vi "IMAQ Readfile.vi"   [LabVIEW 2017]
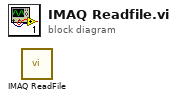
[diagram p0: block diagram]
diagram:
  n1 = call "IMAQ ReadFile"() -> ()  [unwired: 5 in, 7 out]
